vi "input data.vi"(11 "Quantities":T1[](array[typedef])) -> (3 "Quantities out":T1[](array[typedef]))   [LabVIEW 2013]
uses:
  qwtb_lvlib/TD Quantity.ctl
  <vilib>/Utility/xml.llb/Write to XML File(string).vi
  <vilib>/Utility/xml.llb/Read From XML File(string).vi
panel:
  in  "load Q":bool
  in  "save Q":bool
  in  "Q list curr value":i32
  in  "Q list":i32(listbox) caption="Input Quantities"
  in  "quit":bool
  in  "Q name":string caption="Name of Quantity:"
  in  "Q type":enum32{"Scalar", "Vector"}(tab)
  in  "scalar dof":dbl=1.0 caption="DoF"
  in  "scalar value":dbl=1.0 caption="Value"
  in  "scalar unc":dbl=1.0 caption="Uncertainty"
  in  "set dof same as 1st":bool
  in  "vector dof":dbl[](array[numeric]) caption="DoF"
  in  "vector value":dbl[](array[numeric]) caption="Value"
  in  "vector unc":dbl[](array[numeric]) caption="Uncertainty"
  out "Value Graph":dbl[](graph)
  in  "load csv":bool
  in  "set unc same as 1st":bool
  in  "remove Q":bool
  in  "add Q":bool
  # "Input Data"
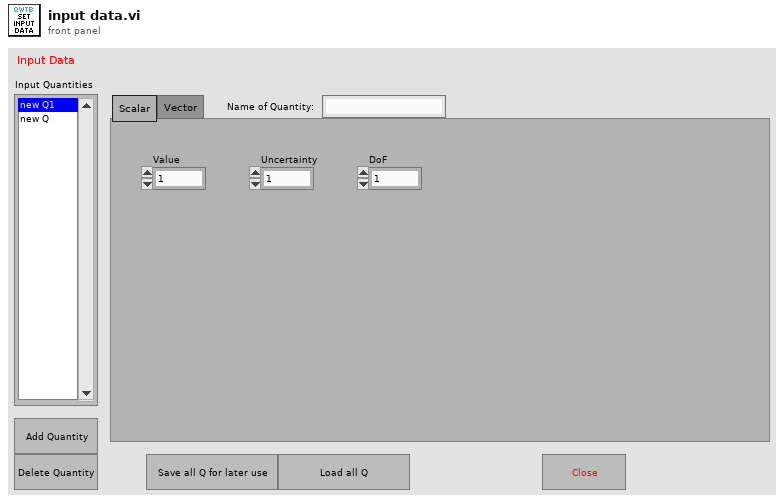
[diagram p1: front panel]
types:
  T1 = typedef "TD Quantity.ctl" = cluster{"Name":string, "Value":dbl[], "Uncertainty":dbl[][], "Degrees of\nFreedom":dbl[]}
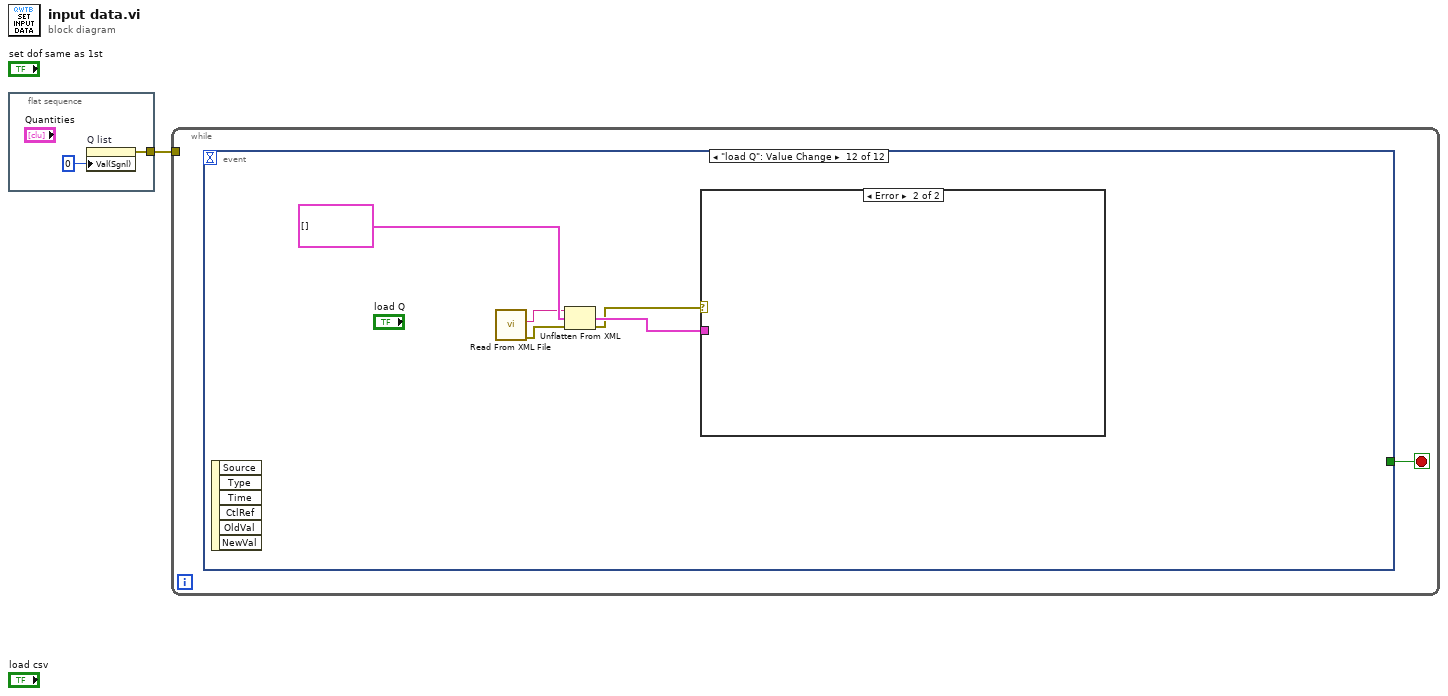
[diagram p0: block diagram]
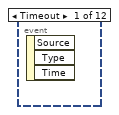
[diagram p2: hidden frame]
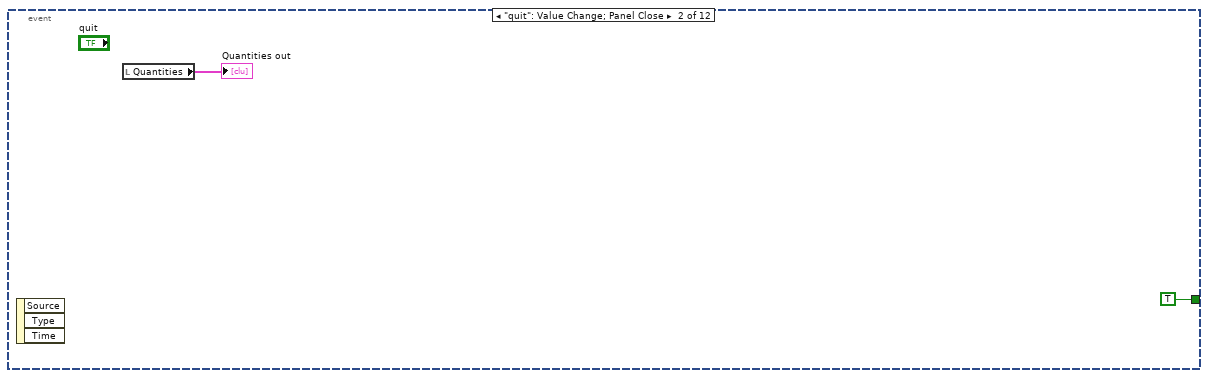
[diagram p3: hidden frame]
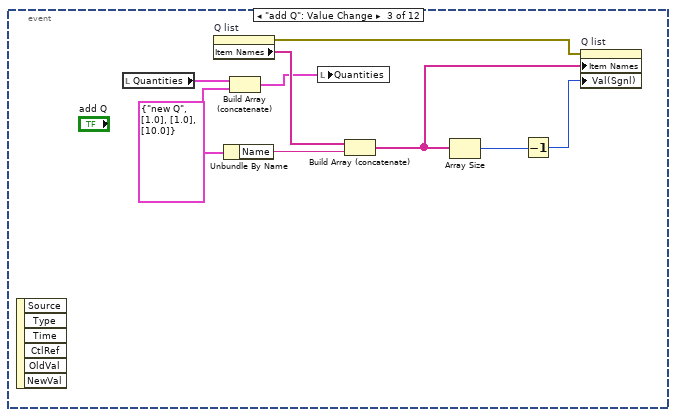
[diagram p4: hidden frame]
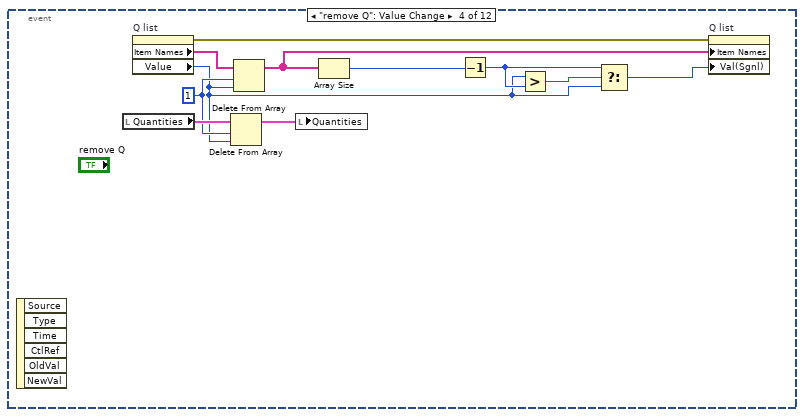
[diagram p5: hidden frame]
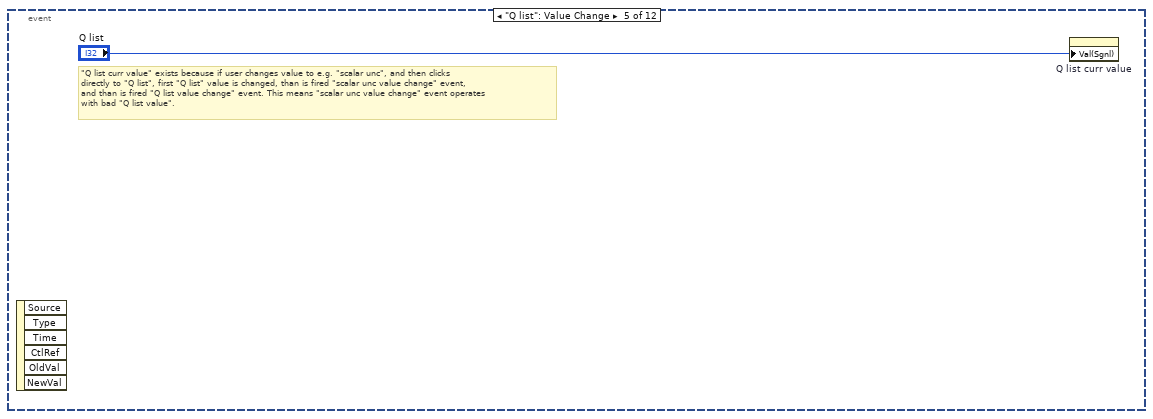
[diagram p6: hidden frame]
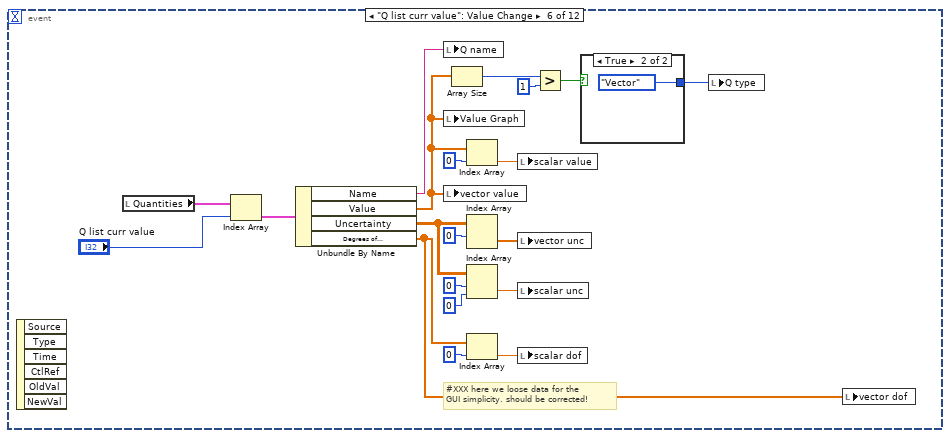
[diagram p7: hidden frame]
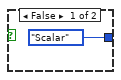
[diagram p8: hidden frame]
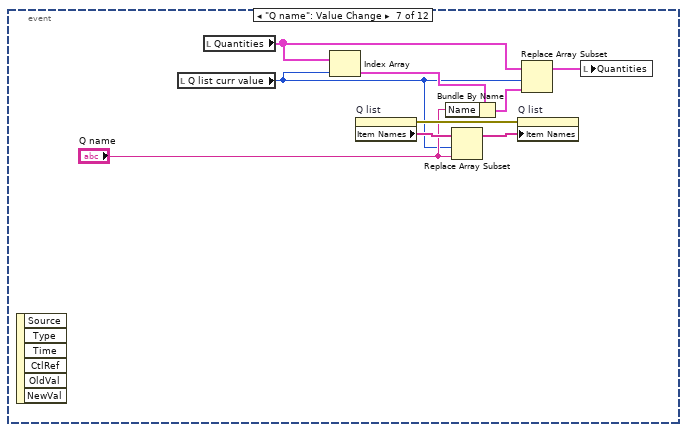
[diagram p9: hidden frame]
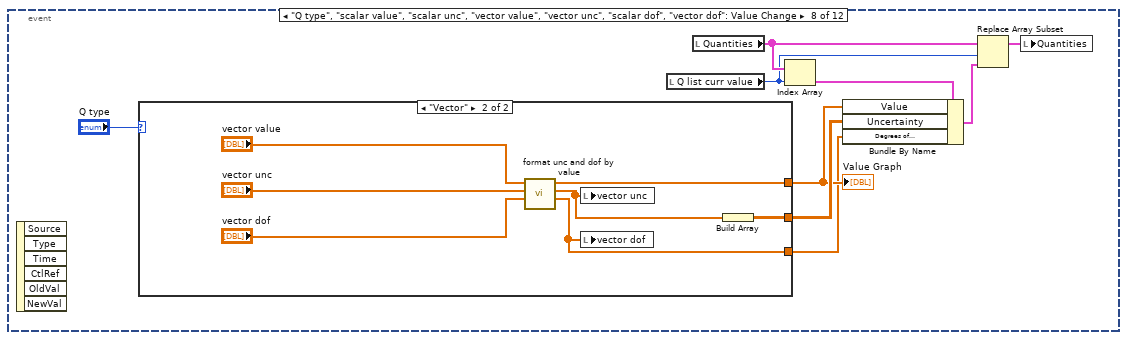
[diagram p10: hidden frame]
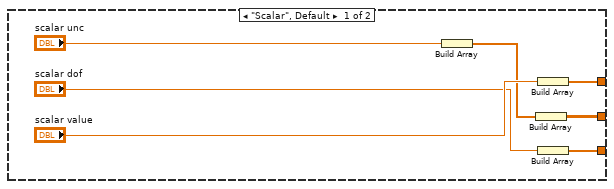
[diagram p11: hidden frame]
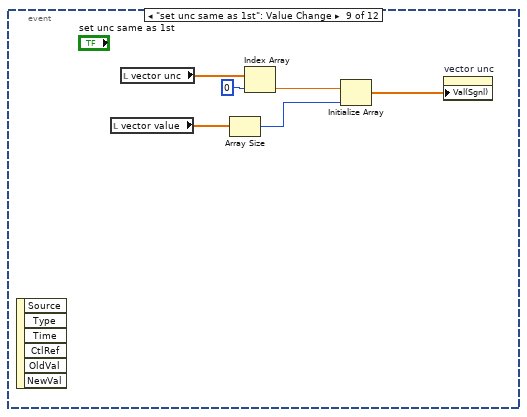
[diagram p12: hidden frame]
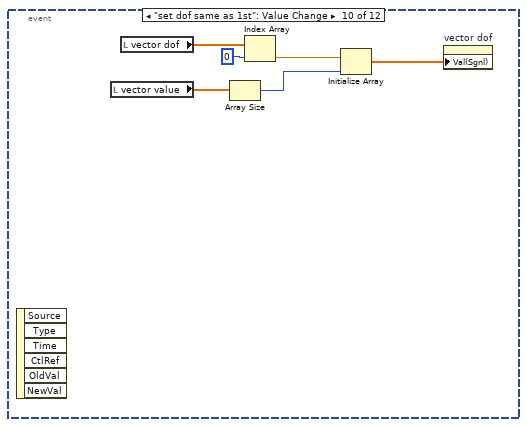
[diagram p13: hidden frame]
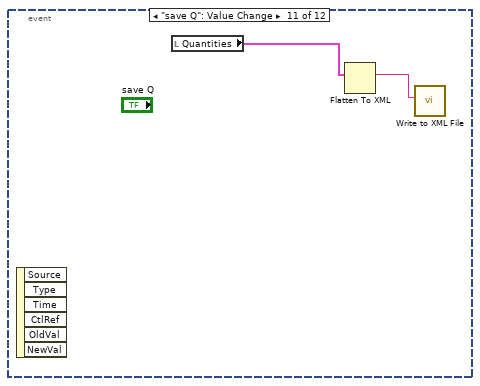
[diagram p14: hidden frame]
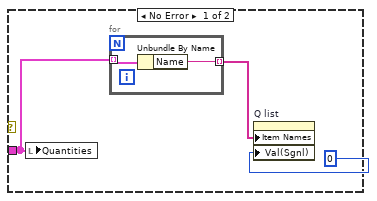
[diagram p15: hidden frame]
diagram:
  n1 = flat-sequence {
    tunnel: [w2] -> w1
    frame #0 {
      n2 = property on="Q list" class="LstBox (strict)"("Val(Sgnl)"=0 ("Value (Signaling)")) -> (error out=w2:errorcluster)  [unwired: 2 in, 1 out]
    }
  }
  n3 = while {
    tunnel: w1 -> [_]
    stop <- w4 stop-if-true
    n4 = event shown="[11] \"load Q\": Value Change" {
      selector: _ -> [_ _ _ _ _ _ _ _ _ _ _ _]
      dyn-events: _ -> [_ _ _ _ _ _ _ _ _ _ _ _]
      timeout: _ -> [_ _ _ _ _ _ _ _ _ _ _ _]
      tunnel: [_ TRUE _ _ _ _ _ _ _ _ _ _] -> w4
      event Timeout {
        n5 = event-data() -> ()  [unwired: 1 in, 3 out]
      }
      event "quit": Value Change; Panel Close {
        n6 = event-data() -> ()  [unwired: 1 in, 3 out]
        n7 = local read "Quantities"() -> (→"Quantities out":T1[])
      }
      event "add Q": Value Change {
        w7 = T1 {"Name"="new Q", "Value"=[1.0], "Uncertainty"=[[1.0]], "Degrees of\nFreedom"=[10.0]} ("Quantity")
        n8 = event-data() -> ()  [unwired: 1 in, 6 out]
        n9 = local read "Quantities"() -> (w10:T1[])
        n10 = property on="Q list" class="LstBox (strict)"() -> (error out=w14:errorcluster, "Item Names"=w15:string[])  [unwired: 2 in, 1 out]
        n11 = Unbundle By Name(w7) -> ("Name"=w8:string)
        n12 = Build Array (concatenate)(w10, w7) -> (w9:T1[])
        n13 = local write "Quantities"(w9) -> ()
        n14 = Build Array (concatenate)(w15, w8) -> (w13:string[])
        n15 = Array Size(array=w13) -> (size(s)=w12:i32)
        n16 = Decrement(x=w12) -> (x-1=w11:i32)
        n17 = property on="Q list" class="LstBox (strict)"(error in=w14, "Item Names"=w13, "Val(Sgnl)"=w11) -> ()  [unwired: 1 in, 2 out]
      }
      event "remove Q": Value Change {
        w18 = 1 ("length")
        n18 = event-data() -> ()  [unwired: 1 in, 6 out]
        n19 = local read "Quantities"() -> (w19:T1[])
        n20 = property on="Q list" class="LstBox (strict)"() -> (error out=w26:errorcluster, "Item Names"=w25:string[], "Value"=w17:i32)  [unwired: 2 in, 1 out]
        n21 = Delete From Array(array=w19, length=w18, index=w17) -> (array with subset deleted=w16:T1[])  [unwired: 1 out]
        n22 = Delete From Array(array=w25, length=w18, index=w17) -> (array with subset deleted=w24:string[])  [unwired: 1 out]
        n23 = local write "Quantities"(w16) -> ()
        n24 = Array Size(array=w24) -> (size(s)=w23:i32)
        n25 = Decrement(x=w23) -> (x-1=w21:i32)
        n26 = Greater?(x=w17, y=w21) -> (0:w22:bool)
        n27 = Select(t=w21, s=w22, f=w17) -> (s? t:f=w20:i32)
        n28 = property on="Q list" class="LstBox (strict)"(error in=w26, "Item Names"=w24, "Val(Sgnl)"=w20) -> ()  [unwired: 1 in, 2 out]
      }
      event "Q list": Value Change {
        # "\"Q list curr value\" exists because if user changes value to e.g. \"scalar unc\", and then clicks\ndirectly to \"Q list\", first \"Q list\" value is changed, than is fired \"scalar unc value change\" event,\nand than is fired \"Q list value change\" event. This means \"scalar unc value change\" event operates\nwith bad \"Q list value\"."
        n29 = event-data() -> ()  [unwired: 1 in, 6 out]
        n30 = property on="Q list curr value" class="DigNum (strict)"("Val(Sgnl)"="Q list") -> ()  [unwired: 2 in, 2 out]
      }
      event "Q list curr value": Value Change {
        # "#XXX here we loose data for the\nGUI simplicity. should be corrected!"
        n31 = event-data() -> ()  [unwired: 1 in, 6 out]
        n32 = local read "Quantities"() -> (w45:T1[])
        n33 = Index Array(array=w45, index="Q list curr value") -> (element=w47:T1)
        n34 = Unbundle By Name(w47) -> ("Name"=w46:string, "Value"=w31:dbl[], "Uncertainty"=w32:dbl[][], "Degrees of\nFreedom"=w28:dbl[])
        n35 = local write "Q name"(w46) -> ()
        n36 = local write "Value Graph"(w31) -> ()
        n37 = local write "vector value"(w31) -> ()
        n38 = Array Size(array=w31) -> (size(s)=w44:i32)
        n39 = Index Array(array=w31, index=0) -> (element=w33:dbl)
        n40 = Index Array(array=w32, index (row)=0) -> (element=w39:dbl[])  [unwired: 1 in]
        n41 = Index Array(array=w32, index (row)=0, index (col)=0 ("disabled index (col)")) -> (element=w36:dbl)
        n42 = Index Array(array=w28, index=0) -> (element=w29:dbl)
        n43 = local write "scalar value"(w33) -> ()
        n44 = local write "vector unc"(w39) -> ()
        n45 = local write "scalar unc"(w36) -> ()
        n46 = local write "scalar dof"(w29) -> ()
        n47 = Greater?(x=w44, y=1) -> (0:w42:bool)
        n48 = case shown="True" w42 {
          tunnel: [enum32{"Scalar", "Vector"}."Scalar" ("Quantity type") enum32{"Scalar", "Vector"}."Vector" ("Quantity type")] -> w41
          frame False {
          }
          frame True {
          }
        }
        n49 = local write "Q type"(w41) -> ()
        n50 = local write "vector dof"(w28) -> ()
      }
      event "Q name": Value Change {
        n51 = event-data() -> ()  [unwired: 1 in, 6 out]
        n52 = local read "Q list curr value"() -> (w51:i32)
        n53 = local read "Quantities"() -> (w57:T1[])
        n54 = Index Array(array=w57, index=w51) -> (element=w58:T1)
        n55 = property on="Q list" class="LstBox (strict)"() -> (error out=w54:errorcluster, "Item Names"=w53:string[])  [unwired: 2 in, 1 out]
        n56 = Bundle By Name(cluster=w58, "Name"="Q name") -> (w56:T1)
        n57 = Replace Array Subset(array=w53, new element="Q name", index=w51) -> (w50:string[])
        n58 = property on="Q list" class="LstBox (strict)"(error in=w54, "Item Names"=w50) -> ()  [unwired: 1 in, 2 out]
        n59 = Replace Array Subset(array=w57, new element=w56, index=w51) -> (w55:T1[])
        n60 = local write "Quantities"(w55) -> ()
      }
      event "Q type", "scalar value", "scalar unc", "vector value", "vector unc", "scalar dof", "vector dof": Value Change {
        n61 = event-data() -> ()  [unwired: 1 in, 6 out]
        n62 = case shown="\"Vector\"" "Q type" {
          tunnel: [w72 w77] -> w60
          tunnel: [w70 w81] -> w66
          tunnel: [w68 w75] -> w59
          frame "Scalar", Default {
            n63 = Build Array("scalar unc") -> (w71:dbl[])
            n64 = Build Array(w71) -> (w70:dbl[][])
            n65 = Build Array("scalar value") -> (w72:dbl[])
            n66 = Build Array("scalar dof") -> (w68:dbl[])
          }
          frame "Vector" {
            n67 = call "format unc and dof by value.vi"("vector dof"="vector dof", "vector unc"="vector unc", "vector value"="vector value") -> ("vector dof out"=w75:dbl[], "vector unc out"=w76:dbl[], "vector value out"=w77:dbl[])  [unwired: 6 in]
            n68 = local write "vector unc"(w76) -> ()
            n69 = local write "vector dof"(w75) -> ()
            n70 = Build Array(w76) -> (w81:dbl[][])
          }
        }
        "Value Graph" <- w60
        n71 = local read "Q list curr value"() -> (w61:i32)
        n72 = local read "Quantities"() -> (w65:T1[])
        n73 = Index Array(array=w65, index=w61) -> (element=w67:T1)
        n74 = Bundle By Name(cluster=w67, "Value"=w60, "Uncertainty"=w66, "Degrees of\nFreedom"=w59) -> (w64:T1)
        n75 = Replace Array Subset(array=w65, new element=w64, index=w61) -> (w63:T1[])
        n76 = local write "Quantities"(w63) -> ()
      }
      event "set unc same as 1st": Value Change {
        n77 = event-data() -> ()  [unwired: 1 in, 6 out]
        n78 = local read "vector value"() -> (w84:dbl[])
        n79 = local read "vector unc"() -> (w87:dbl[])
        n80 = Array Size(array=w84) -> (size(s)=w83:i32)
        n81 = Index Array(array=w87, index=0) -> (element=w85:dbl)
        n82 = Initialize Array(w85, w83) -> (w82:dbl[])
        n83 = property on="vector unc" class="Arr (strict)"("Val(Sgnl)"=w82) -> ()  [unwired: 2 in, 2 out]
      }
      event "set dof same as 1st": Value Change {
        n84 = event-data() -> ()  [unwired: 1 in, 6 out]
        n85 = local read "vector value"() -> (w90:dbl[])
        n86 = local read "vector dof"() -> (w93:dbl[])
        n87 = Array Size(array=w90) -> (size(s)=w89:i32)
        n88 = Index Array(array=w93, index=0) -> (element=w91:dbl)
        n89 = Initialize Array(w91, w89) -> (w88:dbl[])
        n90 = property on="vector dof" class="Arr (strict)"("Val(Sgnl)"=w88) -> ()  [unwired: 2 in, 2 out]
      }
      event "save Q": Value Change {
        n91 = event-data() -> ()  [unwired: 1 in, 6 out]
        n92 = local read "Quantities"() -> (w95:T1[])
        n93 = Flatten To XML(anything=w95) -> (xml string=w94:string)
        n94 = call-poly <vilib>:"Write to XML File.vi"("XML Input"=w94) -> ()  [unwired: 8 in, 3 out]
      }
      event "load Q": Value Change {
        n95 = event-data() -> ()  [unwired: 1 in, 6 out]
        n96 = call-poly <vilib>:"Read From XML File.vi"() -> ("error out"=w100:errorcluster, "XML Elements"=w98:string)  [unwired: 9 in, 1 out]
        n97 = Unflatten From XML(xml string=w98, type=T1[] [], error in (no error)=w100) -> (value=w97:T1[], error out=w96:errorcluster)
        n98 = case shown="Error" w96 {
          tunnel: w97 -> [w103 _]
          frame No Error {
            n99 = local write "Quantities"(w103) -> ()
            n100 = for {
              tunnel: w103 -> [w105] mode=indexing
              tunnel: [w104] -> w101 mode=indexing
              n101 = Unbundle By Name(w105) -> ("Name"=w104:string)
            }
            n102 = property on="Q list" class="LstBox (strict)"("Item Names"=w101, "Val(Sgnl)"=0 ("Value (Signaling)")) -> ()  [unwired: 2 in, 2 out]
          }
          frame Error {
          }
        }
      }
    }
  }
